vi "Configure Acquisition.vi"(4 "Scale / Division (10 dB)":dbl=10.0, 6 "Vertical Scale (0: Linear)":i32(ring) items=["Linear", "Logarithmic"], 7 "Enable Continuous Sweep Mode (F: Disable)":bool, 8 "error in (no error)":errorcluster, 9 "Manual Detector Type (0: Average)":i32(ring) items=["Average", "Peak", "Sample", "Negative peak", "Quasi Peak", "EMI Average", "EMI Peak", "MIL Peak", "RMS"], 10 "Enable Auto Detector (T: Enable)":bool=TRUE, 11 "VISA resource name":refnum<visa-resource-name>) -> (0 "error out":errorcluster, 3 "VISA resource name out":refnum<visa-resource-name>)   [LabVIEW 2014, in "Agilent ESA PSA Series.lvlib"]
doc: "Configures the acquisition properties of the spectrum analyzer."
uses:
  Agilent ESA PSA Series.lvlib
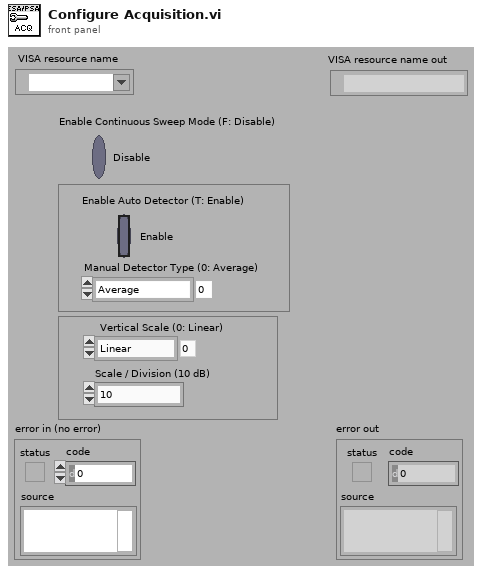
[diagram p1: front panel]
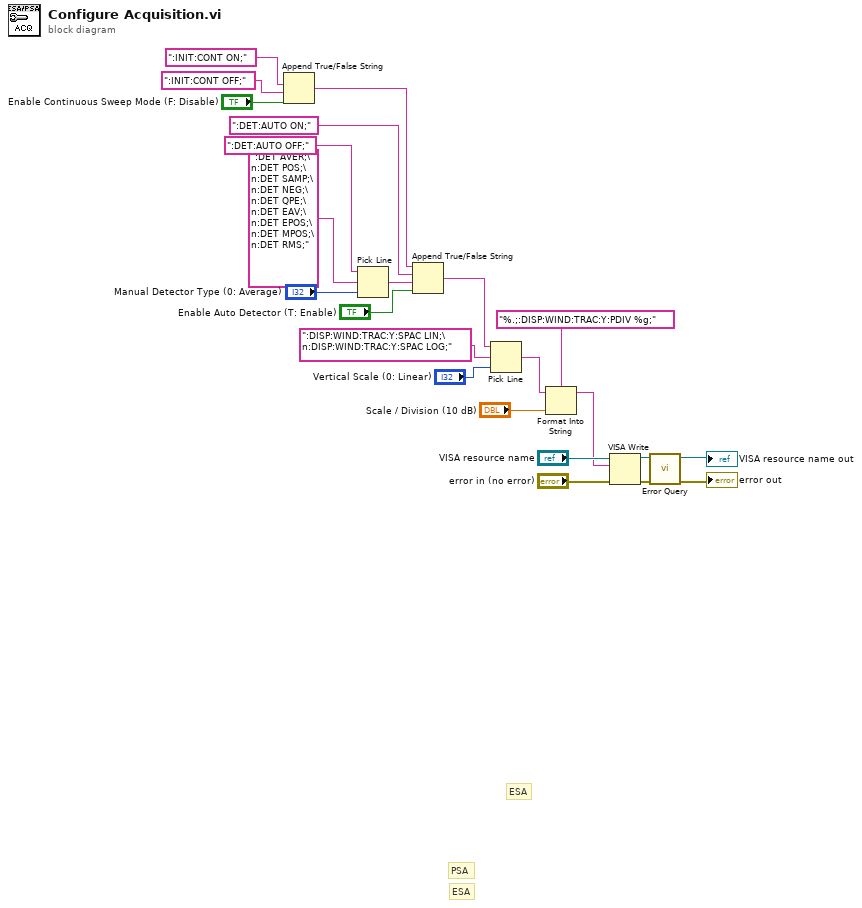
[diagram p0: block diagram]
diagram:
  # "ESA"
  # "PSA"
  # "ESA"
  n1 = Append True/False String(1:"Enable Continuous Sweep Mode (F: Disable)", 2:":INIT:CONT OFF;" ("string (\"\")"), 3:":INIT:CONT ON;" ("string (\"\")")) -> (0:w10:string)  [unwired: 1 in]
  n2 = Pick Line(string ("")=":DET:AUTO OFF;", multi-line string=":DET AVER;\n:DET POS;\n:DET SAMP;\n:DET NEG;\n:DET QPE;\n:DET EAV;\n:DET EPOS;\n:DET MPOS;\n:DET RMS;" ("string (\"\")"), line index="Manual Detector Type (0: Average)") -> (output string=w13:string)
  n3 = Append True/False String(1:"Enable Auto Detector (T: Enable)", 2:w13, 3:":DET:AUTO ON;" ("string (\"\")"), 4:w10) -> (0:w3:string)
  n4 = Pick Line(string ("")=w3, multi-line string=":DISP:WIND:TRAC:Y:SPAC LIN;\n:DISP:WIND:TRAC:Y:SPAC LOG;" ("string (\"\")"), line index="Vertical Scale (0: Linear)") -> (output string=w6:string)
  n5 = Format Into String(format string="%.;:DISP:WIND:TRAC:Y:PDIV %g;", initial string=w6, "Scale / Division (10 dB)") -> (resulting string=w4:string)  [unwired: 1 in, 1 out]
  n6 = VISA Write(VISA resource name="VISA resource name", write buffer=w4, error in (no error)="error in (no error)") -> (VISA resource name out=w2:refnum<visa-resource-name>, error out=w1:errorcluster)  [unwired: 1 out]
  n7 = call "Error Query.vi"("error in (no error)"=w1, "VISA resource name"=w2) -> ("error out"=→"error out":errorcluster, "VISA resource name out"=→"VISA resource name out":refnum<visa-resource-name>)  [unwired: 6 in, 2 out]
